vi "Enable Burst.vi"(0 "RedPitaya connection in":refnum<k5>, 3 "Generation (T: Enable)":bool=TRUE, 5 "error in":errorcluster, 8 "Channel #":u16(ring)=1 items=["Channel 1"=1, "Channel 2"=2], 12 "timeout ms (2000)":i32=2000) -> (14 "RedPitaya connection out":refnum<k5>, 19 "error out":errorcluster)   [LabVIEW 2021, in "RedPitaya.lvlib"]
doc: "Enable or disable burst (pulse) mode. Red Pitaya will generate R-times N-periods of signal and then stop. Time between is P."
uses:
  RedPitaya.lvlib
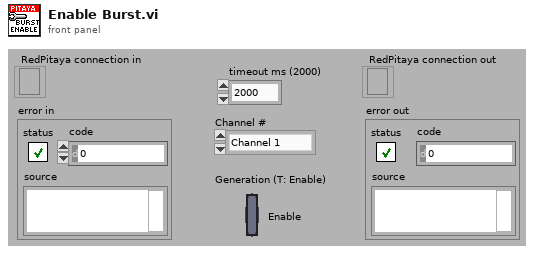
[diagram p1: front panel]
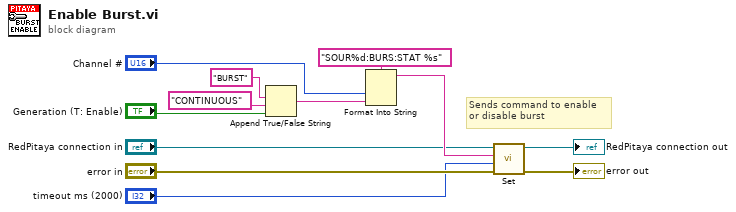
[diagram p0: block diagram]
diagram:
  # "Sends command to enable\nor disable burst"
  n1 = Append True/False String(1:"Generation (T: Enable)", 2:"CONTINUOUS", 3:"BURST") -> (0:w7:string)  [unwired: 1 in]
  n2 = Format Into String(format string="SOUR%d:BURS:STAT %s", "Channel #", w7) -> (resulting string=w6:string)  [unwired: 2 in, 1 out]
  n3 = call "Set.vi"("error in"="error in", "timeout ms (2000)"="timeout ms (2000)", "SCPI Message"=w6, "RedPitaya connection in"="RedPitaya connection in") -> ("error out"=→"error out":errorcluster, "RedPitaya connection out"=→"RedPitaya connection out":refnum<k5>)  [unwired: 5 in, 1 out]
